vi "SimpleExample(MM).vi"() -> ()   [LabVIEW 2020]
uses:
  InstrumentsComm/StellarNet Init & Count.vi
  InstrumentsComm/ReadCoefficients.vi
  Math/Calculate Wavelengths, ext precision.vi
  InstrumentsComm/StellarNet Set Parameters.vi
  InstrumentsComm/StellarNet Scan.vi
  InstrumentsComm/Swdll.dll
panel:
  out "OK":bool
  in  "STOP":bool
  in  "Timeout(Sec)":dbl=1.0 caption="Time Target (s)"
  out "Spectrum":cluster{"Wavelengths":dbl[], "Spectrum":sgl[]}(graph)
  out "Coefficients":dbl[](array[numeric])
  in  "Params":T1={"Integration Time (ms)"=80, "Temp  Compensation "=FALSE, "Optical Smoothing Level"=0, "Number of Scans to Average"=1, "Digitizer Clock Rate Setting"=3} {"Digitizer Clock Rate Setting" min=1 max=3; "Number of Scans to Average" min=1 max=10000 step=1; "Optical Smoothing Level" min=0 max=4 step=1}
  in  "Channel(1)":u32=1 min=1 max=8 step=1
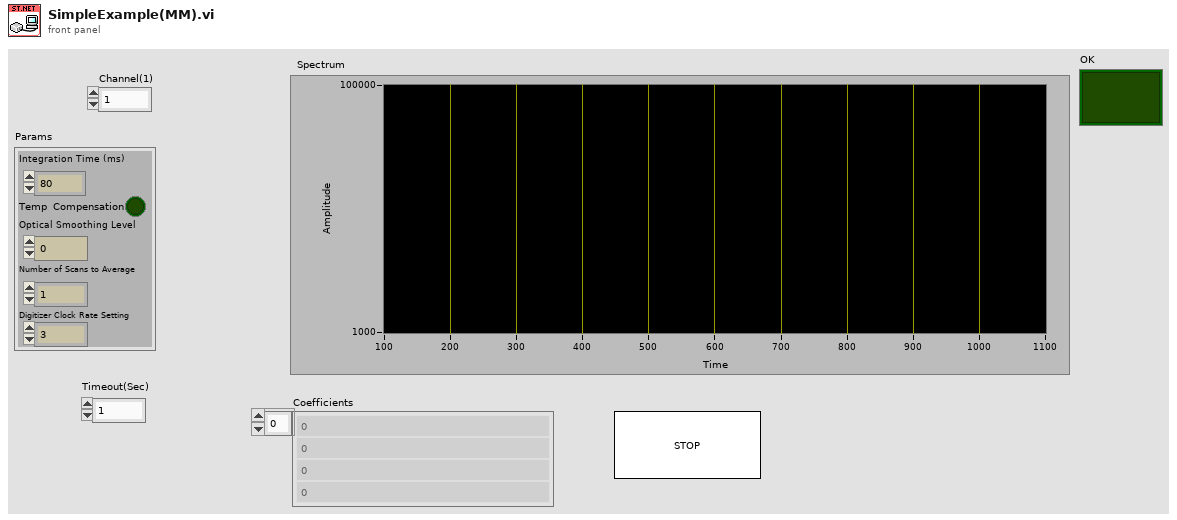
[diagram p1: front panel]
types:
  T1 = cluster{"Integration Time (ms)":i32, "Temp  Compensation ":bool, "Optical Smoothing Level":i32, "Number of Scans to Average":i32, "Digitizer Clock Rate Setting":i32}
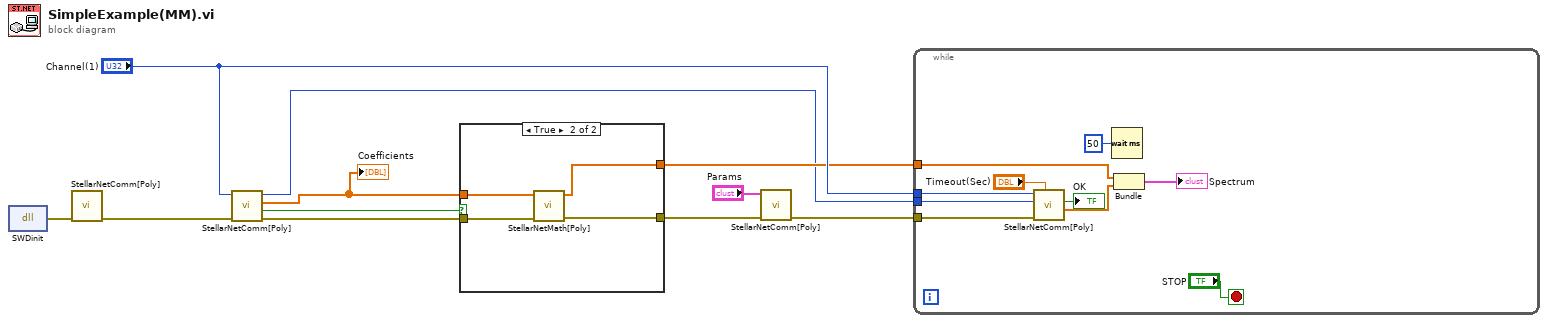
[diagram p0: block diagram]
diagram:
  n1 = dll-call lib="C:/GEECS/Developers Version/source/Device Drivers/StellarNet Black-Comet Spectrometer/SupportLib/InstrumentsComm/swdll.dll" fn="SWDinit" label="init"() -> (error out=w10:errorcluster)  [unwired: 4 in, 1 out]
  n2 = call-poly "StellarNetComm[Poly].vi"("error in"=w10) -> ("error out"=w11:errorcluster)  [unwired: 9 in, 1 out]
  n3 = call-poly "StellarNetComm[Poly].vi"("error in"=w11, "Channel(1)"="Channel(1)") -> ("error out"=w9:errorcluster, "Valid"=w8:bool, "Coefficients"=w2:ext[], "SelectorSpecifier"=w1:u16)  [unwired: 6 in]
  "Coefficients" <- w2
  n4 = case shown="True" w8 {
    tunnel: w9 -> [w12 w16]
    tunnel: w2 -> [_ w15]
    tunnel: [w12 w14] -> w7
    tunnel: [_ w13] -> w4
    frame False {
    }
    frame True {
      n5 = call-poly "StellarNetMath[Poly].vi"("error in"=w16, "C's"=w15) -> ("error out"=w14:errorcluster, "Wavelengths"=w13:dbl[])  [unwired: 8 in]
    }
  }
  n6 = call-poly "StellarNetComm[Poly].vi"("error in"=w7, "Settings"="Params") -> ("error out"=w6:errorcluster)  [unwired: 9 in]
  n7 = while {
    tunnel: w6 -> [w26]
    tunnel: "Channel(1)" -> [w25]
    tunnel: w4 -> [w22]
    tunnel: w1 -> [w17]
    stop <- "STOP" stop-if-true
    n8 = call-poly "StellarNetComm[Poly].vi"("Timeout(Sec)"="Timeout(Sec)", "error in"=w26, "DetectorSpecifier"=w17, "Index"=w25) -> ("Spectrum"=w20:sgl[], "OK"=→"OK":bool)  [unwired: 4 in, 2 out]
    n9 = Wait (ms)(milliseconds to wait=u32 50) -> ()  [unwired: 1 out]
    n10 = Bundle("Wavelengths"=w22, "Spectrum"=w20) -> (→"Spectrum":cluster{"Wavelengths":dbl[], "Spectrum":sgl[]})  [unwired: 1 in]
  }
